vi "写入开始接收数据？.vi"(8 "error in (no error)":errorcluster, 10 "开始接收数据？":bool, 11 "串口通信类 in":refnum<class "串口通信类.lvclass">) -> (0 "error out":errorcluster, 3 "串口通信类 out":refnum<class "串口通信类.lvclass">)   [LabVIEW 2015, in "串口通信类.lvclass"]
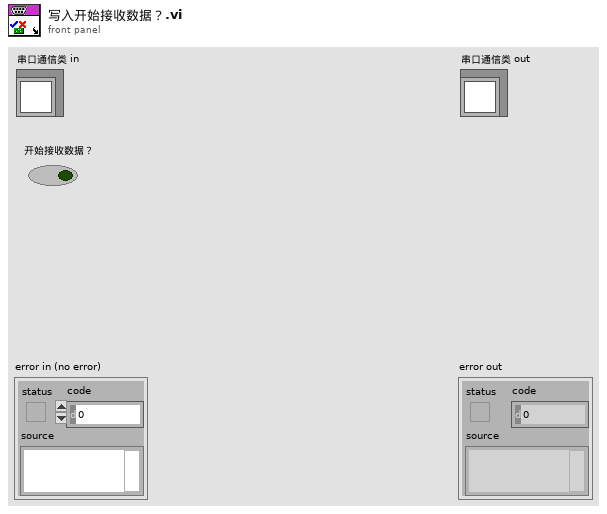
[diagram p1: front panel]
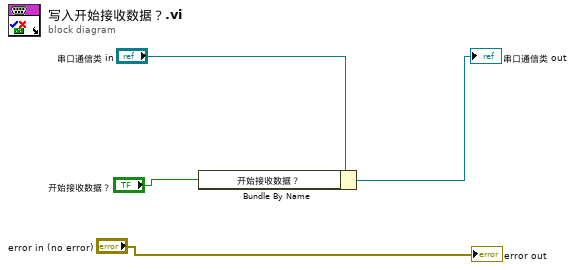
[diagram p0: block diagram]
diagram:
  n1 = Bundle By Name(cluster="串口通信类 in", "开始接收数据？"="开始接收数据？") -> (→"串口通信类 out":refnum<class "串口通信类.lvclass">)
  "error out" <- "error in (no error)"
